vi "Vibrometer Waveforms.vi"() -> ()   [LabVIEW 2025]
uses:
  <vilib>/DAQmx/create/channels.llb/DAQmx Create Channel (AO-Voltage-Basic).vi
  <instrlib>/niScope/Configure/Trigger/niScope Configure Trigger Edge.vi
  <instrlib>/niScope/Configure/Trigger/niScope Configure Trigger Immediate.vi
  <instrlib>/niScope/Acquire/Fetch/niScope Multi Fetch.vi
panel:
  in  "Digitizer Channel":string
  in  "Simulate?":bool
  in  "Data File Name":path
  in  "Data folder Path":path
  out "Filename Out":path
  in  "Min Record Length":i32=1000
  out "Waveform Graph 2":dbl[](graph) caption="averaged wfm"
  in  "Enforce Realtime":bool=TRUE
  out "Waveform Graph 1":dbl[][](graph) caption="Waveform Graph"
  in  "Min. Sample Rate":dbl=1000000.0 format="%#_6p"
  in  "Trigger Type":u16(ring) items=["Edge", "Immediate"]
  in  "Timeout (s)":dbl=5.0 caption="Timeout(s)" format="%.2f"
  in  "Coupling":u16(ring)=1 caption="Trigger Coupling" items=["AC"=0, "DC"=1, "HF Reject"=3, "LF Reject"=4, "AC Plus HF Reject"=1001]
  in  "Trigger Source":string(combo)="0"
  in  "Stop Button":bool
  in  "Vertical Coupling":i32(ring)=1 items=["AC", "DC", "Ground"]
  in  "Num. averages":i32=64
  in  "Resource Name":refnum<k15>="Dev1" caption="Resource Name(s)"
  # "Channels and Destinations"
  # "Configure Parameters"
  # "Constant Parameters"
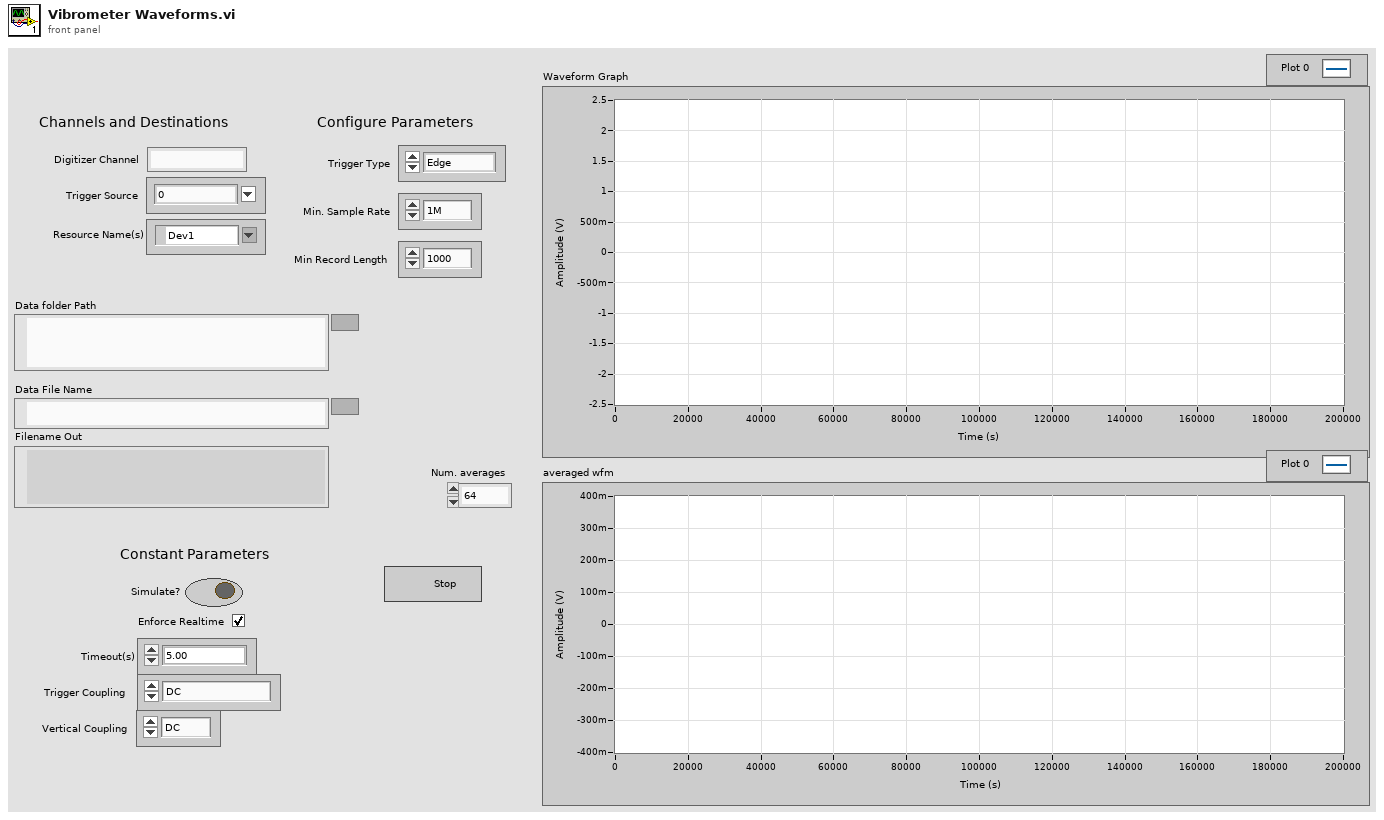
[diagram p1: front panel]
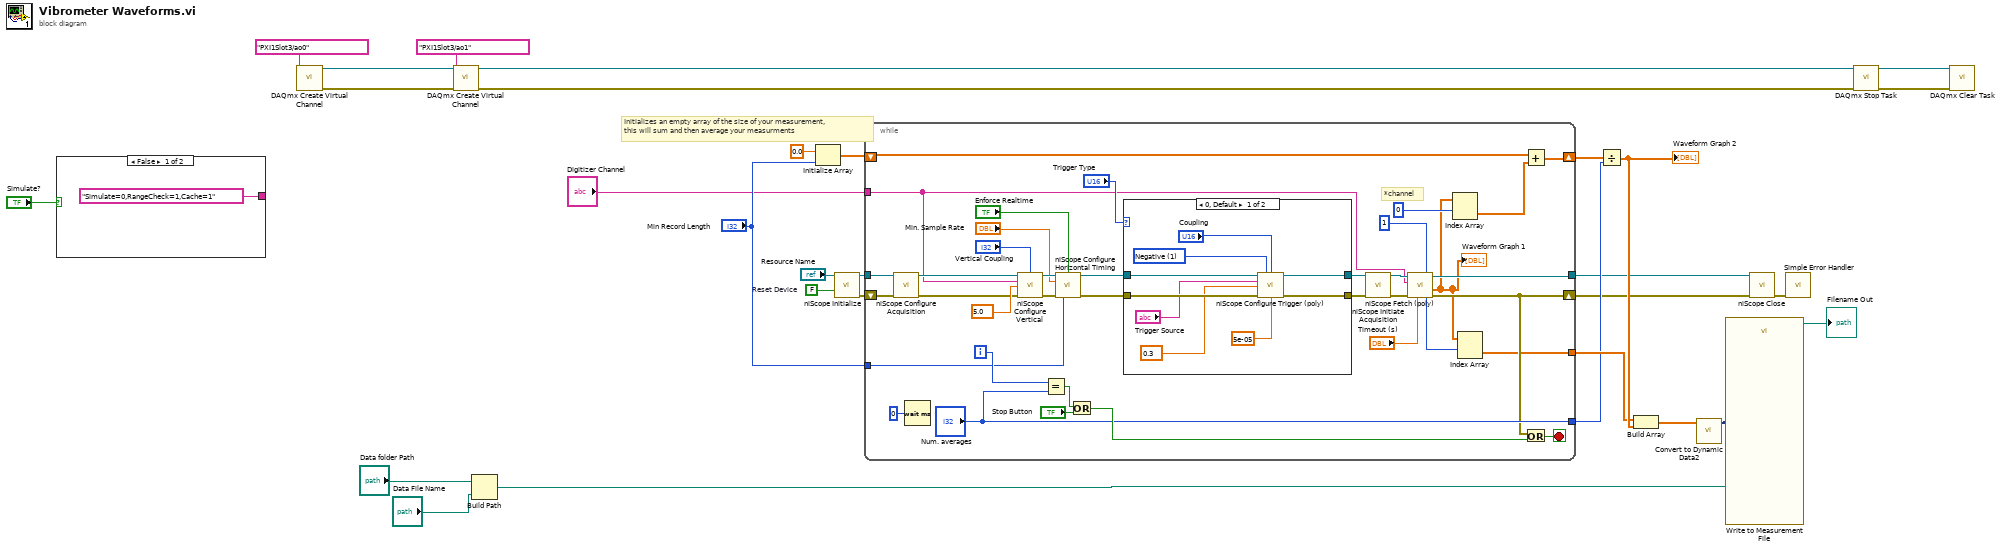
[diagram p0: block diagram]
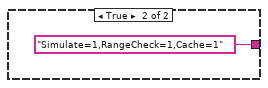
[diagram p2: hidden frame]
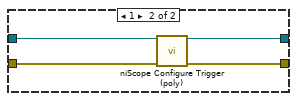
[diagram p3: hidden frame]
diagram:
  w18 = FALSE  # Reset Device
  # "Initializes an empty array of the size of your measurement,\nthis will sum and then average your measurments"
  n1 = case shown="False" "Simulate?" {
    tunnel: ["Simulate=0,RangeCheck=1,Cache=1" ("option string") "Simulate=1,RangeCheck=1,Cache=1" ("option string")] -> _
    frame False {
    }
    frame True {
    }
  }
  n2 = call-poly <vilib>:"DAQmx Create Virtual Channel.vi"("physical channels"=tag "PXI1Slot3/ao0") -> ("task out"=w12:refnum<k21>, "error out"=w11:errorcluster)  [unwired: 13 in]
  n3 = call-poly <vilib>:"DAQmx Create Virtual Channel.vi"("task in"=w12, "physical channels"=tag "PXI1Slot3/ao1", "error in"=w11) -> ("task out"=w3:refnum<k21>, "error out"=w1:errorcluster)  [unwired: 11 in]
  n4 = Build Path(base path="Data folder Path", name or relative path="Data File Name") -> (appended path=w6:path)
  n5 = Initialize Array(0.0 ("element"), "Min Record Length") -> (w25:dbl[])
  n6 = call <instrlib>:"niScope Initialize.vi"("resource name"="Resource Name", "reset device"=w18) -> ("instrument handle"=w21:refnum<k15>, "error out"=w22:errorcluster)  [unwired: 12 in]
  n7 = while {
    tunnel: w21 -> [w56]
    tunnel: [w40] -> w4
    shift-right: [w39] -> w5
    shift-left: w22 -> [w55]
    tunnel: ["Num. averages"] -> w23
    shift-right: [w48] -> w24
    shift-left: w25 -> [w47]
    tunnel: "Min Record Length" -> [w46]
    tunnel: "Digitizer Channel" -> [w41]
    tunnel: [w33] -> w27
    i -> [w50]
    stop <- w57 stop-if-true
    # "*channel"
    n8 = call <instrlib>:"niScope Configure Acquisition.vi"("instrument handle"=w56, "error in"=w55) -> ("instrument handle out"=w62:refnum<k15>, "error out"=w63:errorcluster)  [unwired: 12 in]
    n9 = Wait (ms)(milliseconds to wait=u32 0 ("millisecond multiple")) -> ()  [unwired: 1 out]
    n10 = call <instrlib>:"niScope Configure Vertical.vi"("instrument handle"=w62, "vertical coupling"="Vertical Coupling", "channels"=w41, "vertical range"=5.0 ("Vertical Range (V)"), "error in"=w63) -> ("instrument handle out"=w67:refnum<k15>, "error out"=w68:errorcluster)  [unwired: 9 in]
    n11 = Equal?(x=w50, y="Num. averages") -> (x = y?=w53:bool)
    n12 = call <instrlib>:"niScope Configure Horizontal Timing.vi"("instrument handle"=w67, "enforce realtime"="Enforce Realtime", "min sample rate"="Min. Sample Rate", "error in"=w68, "min record length"=w46) -> ("instrument handle out"=w61:refnum<k15>, "error out"=w60:errorcluster)  [unwired: 9 in]
    n13 = Or(x=w53, y="Stop Button") -> (x .or. y?=w51:bool)
    n14 = case shown="0, Default" "Trigger Type" {
      tunnel: w61 -> [w77 w81]
      tunnel: w60 -> [w76 w78]
      tunnel: [w75 w80] -> w43
      tunnel: [w74 w79] -> w42
      frame 0, Default {
        w72 = u16 1 items=["Positive", "Negative"] ("Trigger Slope")
        n15 = call-poly <instrlib>:"niScope Configure Trigger (poly).vi"("instrument handle"=w77, "trigger slope"=w72, "trigger coupling"="Coupling", "trigger source"="Trigger Source", "trigger level"=0.3 ("Trigger Level"), "error in"=w76, "trigger delay"=5e-05) -> ("instrument handle out"=w75:refnum<k15>, "error out"=w74:errorcluster)  [unwired: 7 in]
      }
      frame 1 {
        n16 = call-poly <instrlib>:"niScope Configure Trigger (poly).vi"("instrument handle"=w81, "error in"=w78) -> ("instrument handle out"=w80:refnum<k15>, "error out"=w79:errorcluster)  [unwired: 12 in]
      }
    }
    n17 = call <instrlib>:"niScope Initiate Acquisition.vi"("instrument handle"=w43, "error in"=w42) -> ("instrument handle out"=w44:refnum<k15>, "error out"=w45:errorcluster)  [unwired: 12 in]
    n18 = call-poly <instrlib>:"niScope Fetch (poly).vi"("timeout"="Timeout (s)", "error in"=w45, "channels"=w41, "instrument handle"=w44) -> ("error out"=w39:errorcluster, "wfm"=w35:dbl[][], "instrument handle out"=w40:refnum<k15>)  [unwired: 4 in, 1 out]
    "Waveform Graph 1" <- w35
    n19 = Index Array(array=w35, index (row)=0) -> (element=w37:dbl[])  [unwired: 1 in]
    n20 = Index Array(array=w35, index (row)=1) -> (element=w33:dbl[])  [unwired: 1 in]
    n21 = Add(x=w47, y=w37) -> (x+y=w48:dbl[])
    n22 = Or(x=w39, y=w51) -> (x .or. y?=w57:bool)
  }
  n23 = Divide(x=w24, y=w23) -> (x/y=w28:dbl[])
  "Waveform Graph 2" <- w28
  n24 = Build Array(w27, w28) -> (w29:dbl[][])
  n25 = call "Convert to Dynamic Data2"("2D Array"=w29) -> ("Dynamic Data Type"=w30:dynamicdata)  [unwired: 3 in]
  n26 = call "Write to Measurement File"("Signals"=w30, "Filename"=w6) -> ("Filename Out"=→"Filename Out":path)  [unwired: 15 in, 2 out]
  n27 = call <instrlib>:"niScope Close.vi"("instrument handle"=w4, "error in"=w5) -> ("error out"=w19:errorcluster)  [unwired: 13 in]
  n28 = call <vilib>:"Simple Error Handler.vi"("error in (no error)"=w19) -> ()  [unwired: 4 in, 5 out]
  n29 = call <vilib>:"DAQmx Stop Task.vi"("task/channels in"=w3, "error in"=w1) -> ("task out"=w16:refnum<k21>, "error out"=w15:errorcluster)  [unwired: 12 in]
  n30 = call <vilib>:"DAQmx Clear Task.vi"("task in"=w16, "error in"=w15) -> ()  [unwired: 13 in, 1 out]
